vi "SetSwerveConfigTrigger.vi"() -> ()   [LabVIEW 2018]
panel:
  in  "rightStickButton":bool=TRUE
  in  "leftStickButton":bool=TRUE
  in  "rightBumper":bool=TRUE
  in  "leftBumper":bool=TRUE
  in  "rightTrigger":dbl format="%#_13g"
  in  "leftTrigget":dbl format="%#_13g"
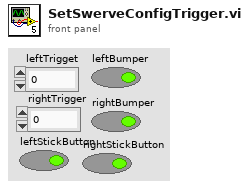
[diagram p1: front panel]
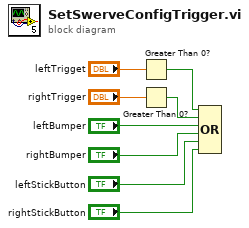
[diagram p0: block diagram]
diagram:
  n1 = Greater Than 0?(x="leftTrigget") -> (x > 0?=w2:bool)
  n2 = Greater Than 0?(x="rightTrigger") -> (x > 0?=w1:bool)
  n3 = Compound Arithmetic op=OR(w2, w1, "leftBumper", "rightBumper", "leftStickButton", "rightStickButton") -> ()  [unwired: 1 out]
